vi "batch action wait on all.vi"() -> ()   [LabVIEW 2015]
uses:
  result/result.lvclass
  standard tasks/batch task/reporting type.ctl
  result/result.lvclass/result.ctl
  result/get data.vi
  result/get error.vi
  result/get owning task.vi
  result/get subresults.vi
  task/task.lvclass
  dispatcher/thread pool.lvclass
  standard reporters/event reporter/event reporter.lvclass
  standard tasks/batch task/batch task.lvclass
  standard action/wait action/wait action.lvclass
panel:
  out "x = y? 2":bool[](array[boolean])
  out "x = y?":bool
  out "owning task":string
  out "error":errorcluster
  out "data":variant
  out "accessors:subresults":refnum<class "result.lvclass">[][](array[class])
  out "owning task":string[](array[string])
  out "Array 2":errorcluster[](array[cluster])
  out "Array":variant[](array[variant])
  out "Time":u32
  out "result":refnum<class "result.lvclass">
  out "error out":errorcluster
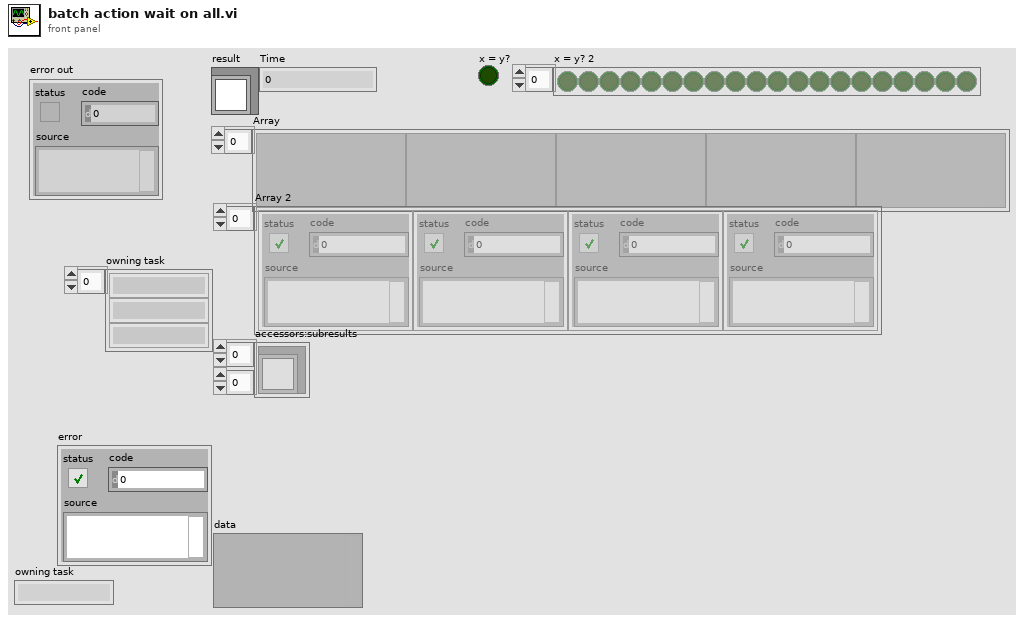
[diagram p1: front panel]
types:
  T1 = typedef "batch task.lvclass/reporting type.ctl" = enum16{"return immediately", "wait on all"}
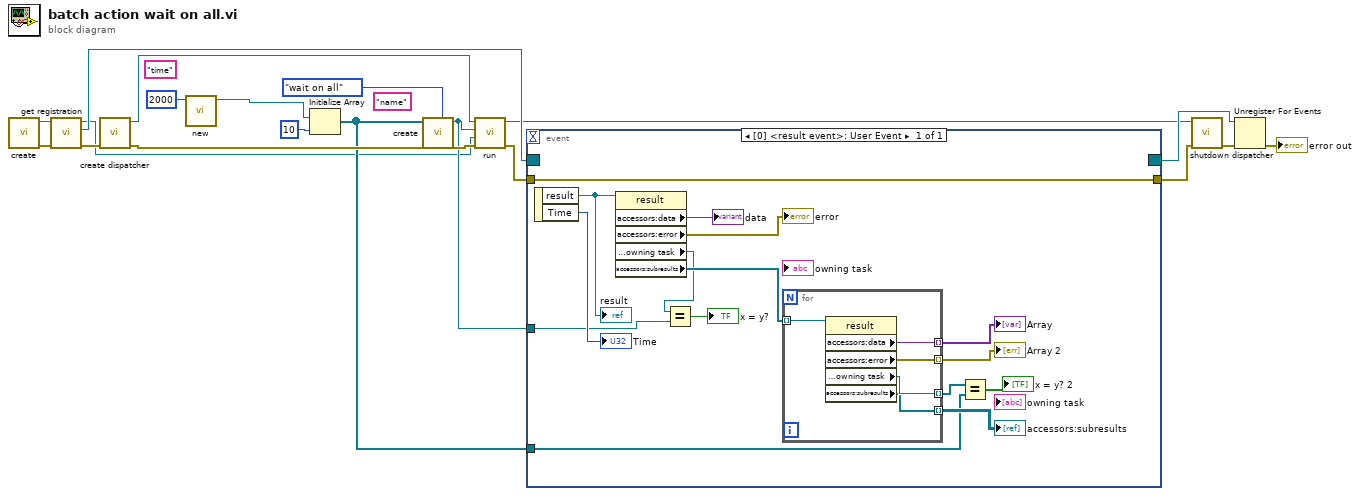
[diagram p0: block diagram]
diagram:
  (unwired) "time" ("ID")
  (unwired) "name" ("ID")
  n1 = call "create.vi"() -> ("error out"=w16:errorcluster, "event reporter out"=w17:refnum<class "event reporter.lvclass">)  [unwired: 10 in]
  n2 = call "get registration.vi"("error in"=w16, "event reporter in"=w17) -> ("error out"=w15:errorcluster, "result registration"=w14:refnum<event-registration>, "event reporter out"=w1:refnum<class "event reporter.lvclass">)  [unwired: 7 in]
  n3 = call "create dispatcher.vi"("error in"=w15) -> ("error out"=w18:errorcluster, "dispatcher"=w19:refnum<class "thread pool.lvclass">)  [unwired: 9 in]
  n4 = call "new.vi"("timer"=2000) -> ("wait action out"=w5:refnum<class "wait action.lvclass">)  [unwired: 10 in]
  n5 = Initialize Array(w5, 10 ("dimension size")) -> (w2:refnum<class "wait action.lvclass">[])
  n6 = call "create.vi"("reporting type"=reporting_type."wait on all", "tasks"=w2) -> ("batch task out"=w3:refnum<class "batch task.lvclass">)  [unwired: 9 in]
  n7 = call "run.vi"("error in"=w18, "results reporter"=w1, "task"=w3, "thread pool in"=w19) -> ("error out"=w8:errorcluster, "thread pool out"=w12:refnum<class "thread pool.lvclass">)  [unwired: 6 in]
  n8 = event shown="[0] <result event>: User Event" {
    selector: w14 -> [_]
    dyn-events: [_] -> w13
    timeout: _ -> [_]
    tunnel: [w33] -> w9
    tunnel: w8 -> [w33]
    tunnel: w3 -> [w24]
    tunnel: w2 -> [w20]
    event User Event {
      n9 = event-data() -> ("result"=w32:refnum<class "result.lvclass">, "Time"=→"Time":u32)  [unwired: 1 in]
      "result" <- w32
      n10 = property class="result"(reference=w32) -> ("accessors:data"=→"data":variant, "accessors:error"=→"error":errorcluster, "accessors:owning task"=w25:refnum<class "task.lvclass">, "accessors:subresults"=w31:refnum<class "result.lvclass">[])  [unwired: 1 in, 2 out]
      n11 = Equal?(x=w25, y=w24) -> (x = y?=→"x = y?":bool)
      n12 = for {
        tunnel: w31 -> [w39] mode=indexing
        tunnel: [w38] -> w30 mode=indexing
        tunnel: [w37] -> w29 mode=indexing
        tunnel: [w36] -> w22 mode=indexing
        tunnel: [w35] -> w28 mode=indexing
        n13 = property class="result"(reference=w39) -> ("accessors:data"=w38:variant, "accessors:error"=w37:errorcluster, "accessors:owning task"=w36:refnum<class "task.lvclass">, "accessors:subresults"=w35:refnum<class "result.lvclass">[])  [unwired: 1 in, 2 out]
      }
      "Array" <- w30
      "Array 2" <- w29
      "accessors:subresults" <- w28
      n14 = Equal?(x=w22, y=w20) -> (x = y?=→"x = y? 2":bool[])
    }
  }
  n15 = call "shutdown dispatcher.vi"("error in"=w9, "thread pool"=w12) -> ("error out"=w11:errorcluster)  [unwired: 9 in]
  n16 = Unregister For Events(event registration refnum=w13, error in=w11) -> (error out=→"error out":errorcluster)
